vi "Host Image Acquisition Loop.vi"(8 "error in":errorcluster) -> (0 "error out":errorcluster)   [LabVIEW 2013]
doc: "Loop handles the image acquisition communication to FPGA.\nInitialize - Queues up the intialize states\n\nExit"
uses:
  Host Image Acquisition Module Enum.ctl
  Message Passing/MsgQ Loops enum.ctl
  Image Acquisition Settings FG Enum.ctl
  System Status/Status FG Enum.ctl
  Globals/Simulation Settings Global.vi
  Common/State Machines/State Machine Lib.lvlib
  Message Passing/Main MsgQ.lvlib
panel:
  out "State":string
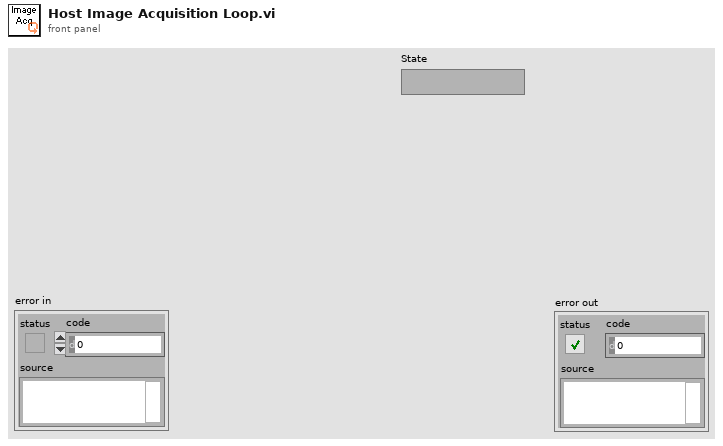
[diagram p1: front panel]
types:
  T1 = typedef "State Machine Lib.lvlib/STATE cluster.ctl" = cluster{"State":string, "Parameters":variant}
  T2 = typedef "Host Image Acquisition Module Enum.ctl" = enum16{"Open FPGA", "Initialize DMA FIFO", "Load Sim Images", "Initialize Acquisition", "Update Sector Parameters", "Start Acquisition", "Aquire Image", "Read Averages", "Cancel Acquisition", "Close FPGA"}
  T3 = typedef "Main MsgQ.lvlib/MsgQ Loops enum.ctl" = enum16{"User Interface", "Image Acq"}
  T4 = typedef "Image Acquisition Settings FG Enum.ctl" = enum16{"Read", "Write"}
  T5 = typedef "Status FG Enum.ctl" = enum16{"Reset", "Read", "Write"}
  T6 = typedef "Simulation Settings Cluster.ctl" = cluster{"Sim Enabled?":bool, "Sim Path":path}
  T7 = typedef "Acquisition Settings Cluster.ctl" = cluster{"Image Width":u32, "Image Height":u32, "Frames To Acquire":u32, "Signal Mapping":enum8{"Standard", "Basler 10-tap", "Vosskühler 10-tap"}, "DMA Buffer Size\n(In Images)":u32}
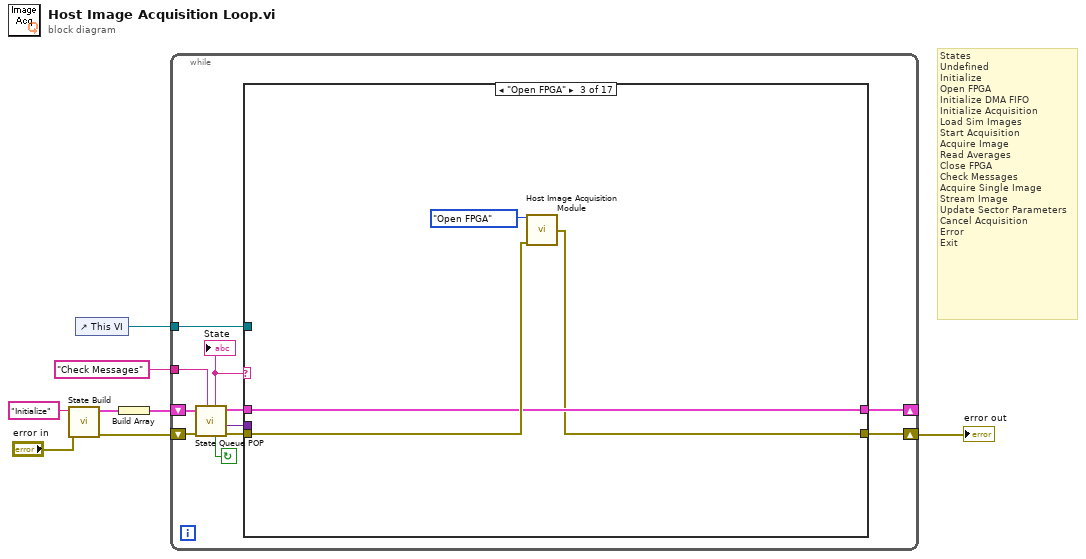
[diagram p0: block diagram]
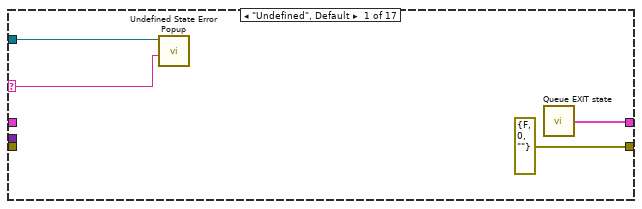
[diagram p2: hidden frame]
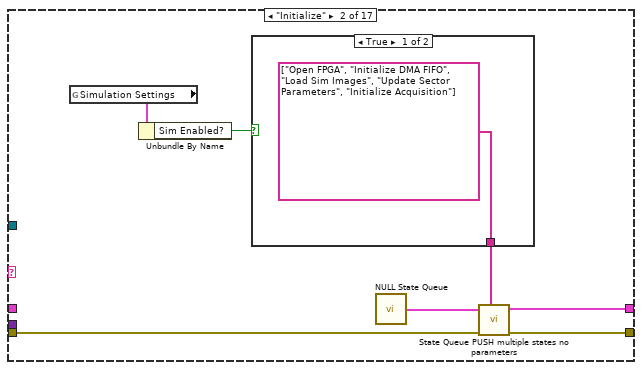
[diagram p3: hidden frame]
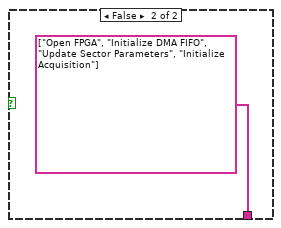
[diagram p4: hidden frame]
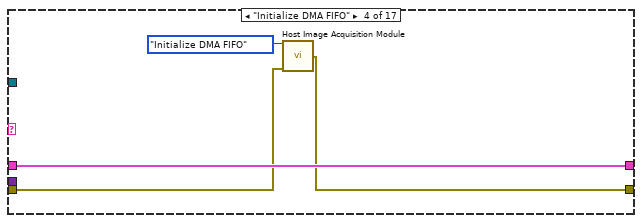
[diagram p5: hidden frame]
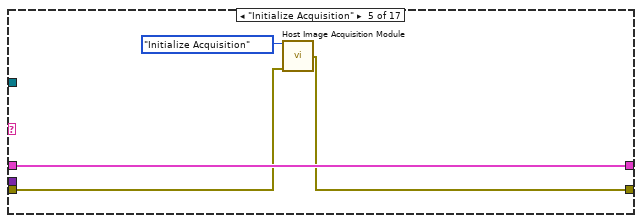
[diagram p6: hidden frame]
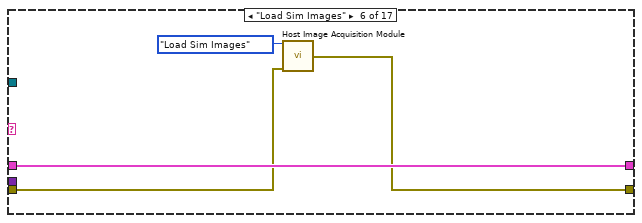
[diagram p7: hidden frame]
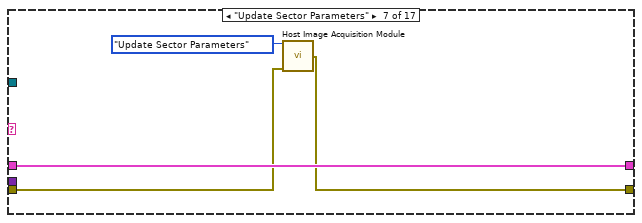
[diagram p8: hidden frame]
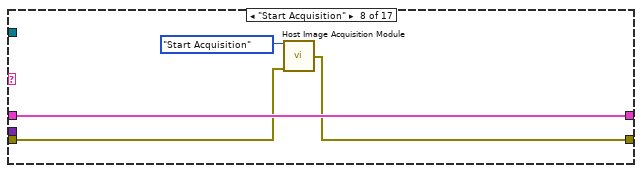
[diagram p9: hidden frame]
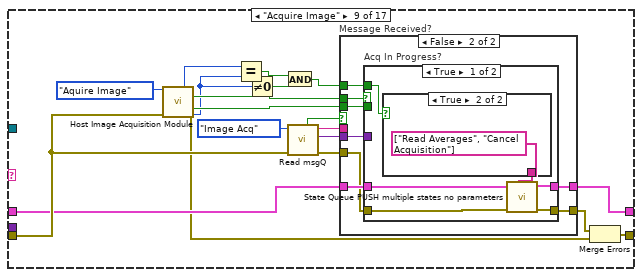
[diagram p10: hidden frame]
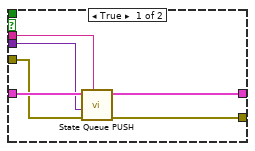
[diagram p11: hidden frame]
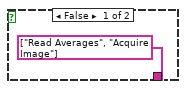
[diagram p12: hidden frame]
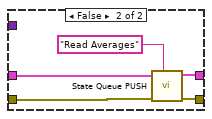
[diagram p13: hidden frame]
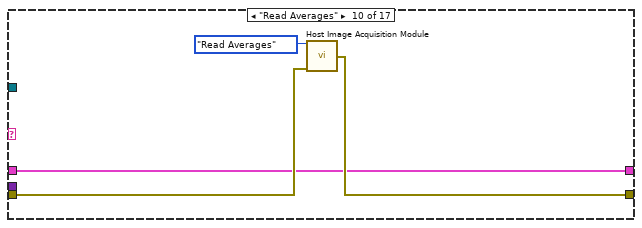
[diagram p14: hidden frame]
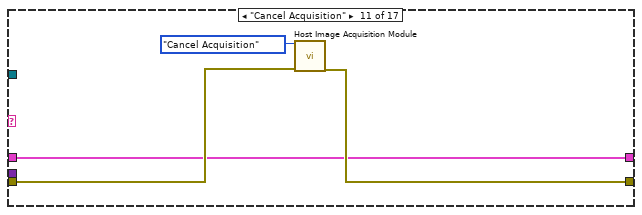
[diagram p15: hidden frame]
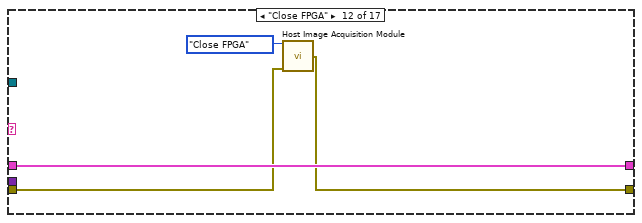
[diagram p16: hidden frame]
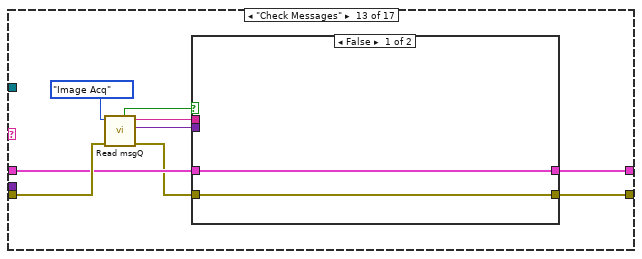
[diagram p17: hidden frame]
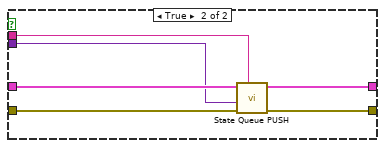
[diagram p18: hidden frame]
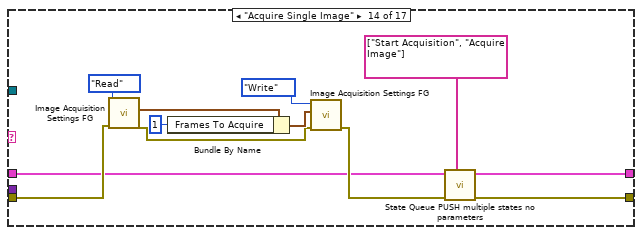
[diagram p19: hidden frame]
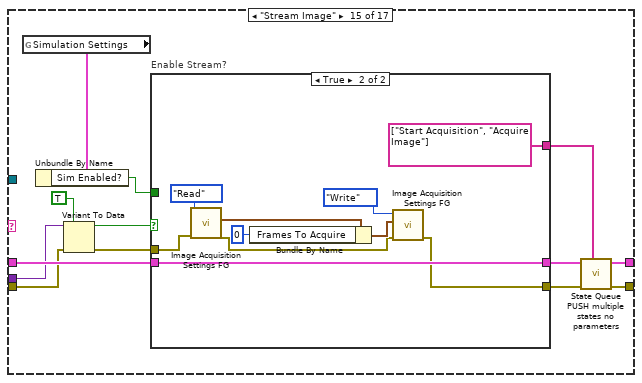
[diagram p20: hidden frame]
diagram:
  # "States\nUndefined\nInitialize\nOpen FPGA\nInitialize DMA FIFO\nInitialize Acquisition\nLoad Sim Images\nStart Acquisition\nAcquire Image\nRead Averages\nClose FPGA\nCheck Messages\nAcquire Single Image\nStream Image\nUpdate Sector Parameters\nCancel Acquisition\nError\nExit"
  n1 = call "State Build.vi"("error in (no error)"="error in", "State"="Initialize") -> ("error out"=w4:errorcluster, "State Out"=w6:T1)  [unwired: 8 in]
  n2 = control-ref of="This VI"() -> (w1:refnum<vi>)
  n3 = Build Array(w6) -> (w5:T1[])
  n4 = while {
    shift-right: [w12] -> _
    shift-left: w5 -> [w19]
    shift-right: [w11] -> w2
    shift-left: w4 -> [w18]
    tunnel: "Check Messages" ("Default state") -> [w16]
    tunnel: w1 -> [w10]
    stop <- w17 continue-if-true
    n5 = call "State Queue POP.vi"("Default state"=w16, "error in (no error)"=w18, "State que in"=w19) -> ("error out"=w13:errorcluster, "Parameters"=w9:variant, "State que out"=w14:T1[], "Not Exit?"=w17:bool, "State case out"=w15:string)  [unwired: 4 in]
    "State" <- w15
    n6 = case shown="\"Open FPGA\"" w15 {
      selector: w15 -> [w22 _ _ _ _ _ _ _ _ _ _ _ _ _ _ _ _]
      tunnel: w14 -> [_ _ w34 w40 w44 w48 w52 w56 w73 w103 w107 w114 w121 w135 w156 w172 w179]
      tunnel: w13 -> [_ w30 w35 w39 w43 w47 w51 w55 w74 w105 w109 w113 w123 w142 w146 w175 w178]
      tunnel: [w21 w27 w34 w40 w44 w48 w52 w56 w72 w103 w107 w114 w120 w133 w151 w172 w179] -> w12
      tunnel: [errorcluster {"status"=FALSE, "code"=0, "source"=""} ("error out") w26 w33 w38 w42 w45 w50 w54 w70 w104 w108 w112 w119 w132 w149 w173 w178] -> w11
      tunnel: w10 -> [w23 _ _ _ _ _ _ _ _ _ _ _ _ _ _ _ _]
      tunnel: w9 -> [_ _ _ _ _ _ _ _ _ _ _ _ _ _ w155 _ _]
      frame "Undefined", Default {
        n7 = call "Undefined State Error Popup.vi"("String"=w22, "This VI (Caller if unwired)"=w23) -> ()  [unwired: 10 in]
        n8 = call "Queue EXIT state.vi"() -> ("Exit State Q"=w21:T1[])  [unwired: 1 in]
      }
      frame "Initialize" {
        n9 = global read "Simulation Settings Global.vi" "Simulation Settings"() -> (w25:T6)
        n10 = Unbundle By Name(w25) -> ("Sim Enabled?"=w24:bool)
        n11 = case shown="True" w24 {
          tunnel: [string[] ["Open FPGA", "Initialize DMA FIFO", "Load Sim Images", "Update Sector Parameters", "Initialize Acquisition"] ("States to queue") string[] ["Open FPGA", "Initialize DMA FIFO", "Update Sector Parameters", "Initialize Acquisition"] ("States to queue")] -> w28
          frame True {
          }
          frame False {
          }
        }
        n12 = call "NULL State Queue.vi"() -> ("NULL State Queue"=w29:T1[])
        n13 = call "State Queue PUSH multiple states no parameters.vi"("States to queue"=w28, "error in (no error)"=w30, "State que in"=w29) -> ("error out"=w26:errorcluster, "State que out"=w27:T1[])  [unwired: 7 in]
      }
      frame "Open FPGA" {
        n14 = call "Host Image Acquisition Module.vi"("Operation"=Host_Image_Acquisition_Module_Enum."Open FPGA", "error in"=w35) -> ("error out"=w33:errorcluster)  [unwired: 5 in, 8 out]
      }
      frame "Initialize DMA FIFO" {
        n15 = call "Host Image Acquisition Module.vi"("Operation"=Host_Image_Acquisition_Module_Enum."Initialize DMA FIFO", "error in"=w39) -> ("error out"=w38:errorcluster)  [unwired: 5 in, 8 out]
      }
      frame "Initialize Acquisition" {
        n16 = call "Host Image Acquisition Module.vi"("Operation"=Host_Image_Acquisition_Module_Enum."Initialize Acquisition", "error in"=w43) -> ("error out"=w42:errorcluster)  [unwired: 5 in, 8 out]
      }
      frame "Load Sim Images" {
        n17 = call "Host Image Acquisition Module.vi"("Operation"=Host_Image_Acquisition_Module_Enum."Load Sim Images", "error in"=w47) -> ("error out"=w45:errorcluster)  [unwired: 5 in, 8 out]
      }
      frame "Update Sector Parameters" {
        n18 = call "Host Image Acquisition Module.vi"("Operation"=Host_Image_Acquisition_Module_Enum."Update Sector Parameters", "error in"=w51) -> ("error out"=w50:errorcluster)  [unwired: 5 in, 8 out]
      }
      frame "Start Acquisition" {
        n19 = call "Host Image Acquisition Module.vi"("Operation"=Host_Image_Acquisition_Module_Enum."Start Acquisition", "error in"=w55) -> ("error out"=w54:errorcluster)  [unwired: 5 in, 8 out]
      }
      frame "Acquire Image" {
        n20 = call "Host Image Acquisition Module.vi"("Operation"=Host_Image_Acquisition_Module_Enum."Aquire Image", "error in"=w74) -> ("Num Frames read"=w61:u32, "Acq In Progress"=w69:bool, "error out"=w71:errorcluster, "Image Acquired"=w68:bool, "Frames To Acquire"=w57:u32)  [unwired: 5 in, 4 out]
        n21 = Equal?(x=w61, y=w57) -> (x = y?=w60:bool)
        n22 = Not Equal To 0?(x=w57) -> (x != 0?=w58:bool)
        n23 = And(x=w60, y=w58) -> (x .and. y?=w59:bool)
        n24 = call "Read msgQ.vi"("error in"=w74, "MsgQ enum"=MsgQ_Loops_enum."Image Acq") -> ("error out"=w64:errorcluster, "Message Received Parameters"=w62:variant, "Message Received String"=w65:string, "Message Recieved?"=w66:bool)  [unwired: 6 in]
        n25 = case "Message Received?" shown="False" w66 {
          tunnel: w65 -> [w80 _]
          tunnel: w64 -> [w79 w88]
          tunnel: w73 -> [w81 w89]
          tunnel: [w78 w87] -> w63
          tunnel: [w77 w86] -> w72
          tunnel: w69 -> [_ w85]
          tunnel: w62 -> [w76 w84]
          tunnel: w68 -> [_ w83]
          tunnel: w59 -> [_ w82]
          frame True {
            n26 = call "State Queue PUSH.vi"("State case"=w80, "error in (no error)"=w79, "Parameters"=w76, "State que in"=w81) -> ("error out"=w78:errorcluster, "State que out"=w77:T1[])  [unwired: 6 in]
          }
          frame False {
            n27 = case "Acq In Progress?" shown="True" w85 {
              tunnel: w89 -> [w95 w102]
              tunnel: w88 -> [w92 w99]
              tunnel: [w93 w100] -> w87
              tunnel: [w94 w101] -> w86
              tunnel: w84 -> [_ _]
              tunnel: w83 -> [_ _]
              tunnel: w82 -> [w90 _]
              frame True {
                n28 = case shown="True" w90 {
                  tunnel: [string[] ["Read Averages", "Acquire Image"] ("States to queue") string[] ["Read Averages", "Cancel Acquisition"] ("States to queue")] -> w91
                  frame False {
                  }
                  frame True {
                  }
                }
                n29 = call "State Queue PUSH multiple states no parameters.vi"("States to queue"=w91, "error in (no error)"=w92, "State que in"=w95) -> ("error out"=w93:errorcluster, "State que out"=w94:T1[])  [unwired: 7 in]
              }
              frame False {
                n30 = call "State Queue PUSH.vi"("State case"="Read Averages", "error in (no error)"=w99, "State que in"=w102) -> ("error out"=w100:errorcluster, "State que out"=w101:T1[])  [unwired: 7 in]
              }
            }
          }
        }
        n31 = Merge Errors(w63, w71) -> (w70:errorcluster)
      }
      frame "Read Averages" {
        n32 = call "Host Image Acquisition Module.vi"("Operation"=Host_Image_Acquisition_Module_Enum."Read Averages", "error in"=w105) -> ("error out"=w104:errorcluster)  [unwired: 5 in, 8 out]
      }
      frame "Cancel Acquisition" {
        n33 = call "Host Image Acquisition Module.vi"("Operation"=Host_Image_Acquisition_Module_Enum."Cancel Acquisition", "error in"=w109) -> ("error out"=w108:errorcluster)  [unwired: 5 in, 8 out]
      }
      frame "Close FPGA" {
        n34 = call "Host Image Acquisition Module.vi"("Operation"=Host_Image_Acquisition_Module_Enum."Close FPGA", "error in"=w113) -> ("error out"=w112:errorcluster)  [unwired: 5 in, 8 out]
      }
      frame "Check Messages" {
        n35 = call "Read msgQ.vi"("error in"=w123, "MsgQ enum"=MsgQ_Loops_enum."Image Acq") -> ("error out"=w118:errorcluster, "Message Received Parameters"=w115:variant, "Message Received String"=w117:string, "Message Recieved?"=w122:bool)  [unwired: 6 in]
        n36 = case shown="False" w122 {
          tunnel: w121 -> [w125 w131]
          tunnel: [w125 w130] -> w120
          tunnel: [w124 w129] -> w119
          tunnel: w118 -> [w124 w128]
          tunnel: w117 -> [_ w126]
          tunnel: w115 -> [_ w127]
          frame False {
          }
          frame True {
            n37 = call "State Queue PUSH.vi"("State case"=w126, "error in (no error)"=w128, "Parameters"=w127, "State que in"=w131) -> ("error out"=w129:errorcluster, "State que out"=w130:T1[])  [unwired: 6 in]
          }
        }
      }
      frame "Acquire Single Image" {
        n38 = call "Image Acquisition Settings FG.vi"("error in (no error)"=w142, "Operation"=Image_Acquisition_Settings_FG_Enum."Read") -> ("error out"=w137:errorcluster, "Acquisition Settings Out"=w141:T7)  [unwired: 8 in]
        n39 = Bundle By Name(cluster=w141, "Frames To Acquire"=u32 1) -> (w139:T7)
        n40 = call "Image Acquisition Settings FG.vi"("error in (no error)"=w137, "Acquisition Settings In"=w139, "Operation"=Image_Acquisition_Settings_FG_Enum."Write") -> ("error out"=w136:errorcluster)  [unwired: 7 in, 1 out]
        n41 = call "State Queue PUSH multiple states no parameters.vi"("States to queue"=string[] ["Start Acquisition", "Acquire Image"], "error in (no error)"=w136, "State que in"=w135) -> ("error out"=w132:errorcluster, "State que out"=w133:T1[])  [unwired: 7 in]
      }
      frame "Stream Image" {
        n42 = global read "Simulation Settings Global.vi" "Simulation Settings"() -> (w147:T6)
        n43 = Unbundle By Name(w147) -> ("Sim Enabled?"=w144:bool)
        n44 = Variant To Data(error in=w146, type=TRUE, Variant=w155) -> (data=w153:bool, error out=w145:errorcluster)
        n45 = case "Enable Stream?" shown="True" w153 {
          tunnel: w145 -> [w157 w169]
          tunnel: w156 -> [w158 w168]
          tunnel: [w158 w168] -> w152
          tunnel: [w157 w167] -> w150
          tunnel: [string[] ["Cancel Acquisition"] ("States to queue") string[] ["Start Acquisition", "Acquire Image"] ("States to queue")] -> w148
          tunnel: w144 -> [_ _]
          frame False {
          }
          frame True {
            n46 = call "Image Acquisition Settings FG.vi"("error in (no error)"=w169, "Operation"=Image_Acquisition_Settings_FG_Enum."Read") -> ("error out"=w160:errorcluster, "Acquisition Settings Out"=w164:T7)  [unwired: 8 in]
            n47 = Bundle By Name(cluster=w164, "Frames To Acquire"=u32 0) -> (w162:T7)
            n48 = call "Image Acquisition Settings FG.vi"("error in (no error)"=w160, "Acquisition Settings In"=w162, "Operation"=Image_Acquisition_Settings_FG_Enum."Write") -> ("error out"=w167:errorcluster)  [unwired: 7 in, 1 out]
          }
        }
        n49 = call "State Queue PUSH multiple states no parameters.vi"("States to queue"=w148, "error in (no error)"=w150, "State que in"=w152) -> ("error out"=w149:errorcluster, "State que out"=w151:T1[])  [unwired: 7 in]
      }
      frame "Error" {
        n50 = Unbundle By Name(w175) -> ("source"=w176:string)
        n51 = Concatenate Strings("Error: " ("string"), w176) -> (w171:string)
        n52 = call "Status FG.vi"("Status In"=w171, "Operation"=Status_FG_Enum."Write") -> ()  [unwired: 8 in, 2 out]
        n53 = call "Broadcast Exit.vi"("error in"=errorcluster {"status"=FALSE, "code"=0, "source"=""}) -> ("error out"=w173:errorcluster)  [unwired: 10 in]
      }
      frame "Exit" {
      }
    }
  }
  "error out" <- w2
